vi "Labview to arduino VISA.vi"() -> ()   [LabVIEW 2012]
uses:
  <vilib>/Instr/_visa.llb/VISA Configure Serial Port (Instr).vi
panel:
  out "Meter":dbl(knob) scale=0.0..1024.0
  out "Waveform Chart":dbl(graph)
  out "Extracted Value":dbl
  in  "All Off":bool
  in  "LED 3":bool
  in  "LED 2":bool
  in  "LED 1":bool
  in  "Slide":dbl(slide) step=1.0 scale=0.0..1.0 scale format="%#_1g"
  out "Bytes Read":u32
  out "Raw Output":string="\n"
  in  "Input":refnum<visa-resource-name>="COM1"
  in  "Baud Rate":u32=9600
  # "Read"
  # "Write"
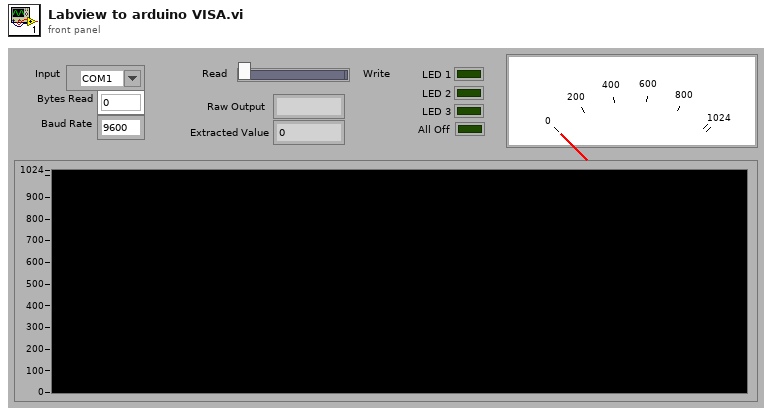
[diagram p1: front panel]
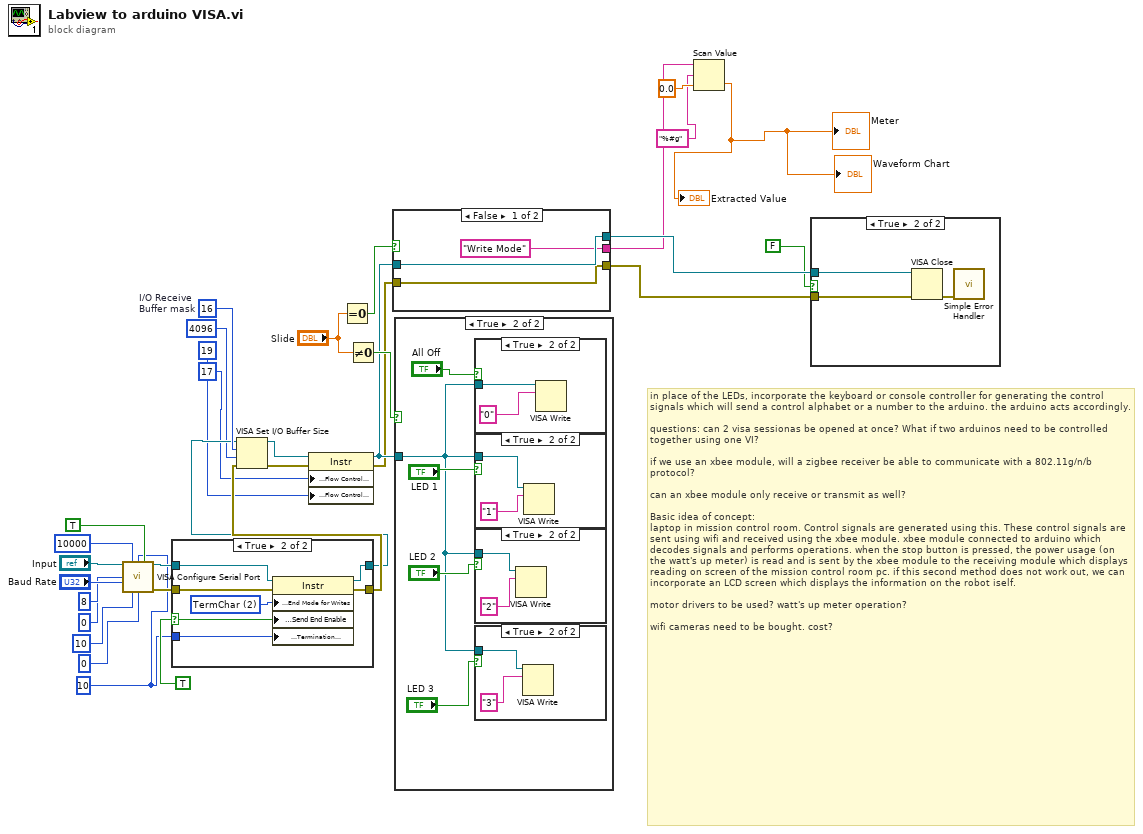
[diagram p0: block diagram]
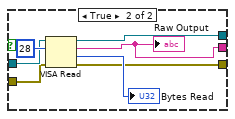
[diagram p8: hidden frame]
diagram:
  w13 = u8 10
  w30 = u16 16  # I/O Receive Buffer mask
  # "in place of the LEDs, incorporate the keyboard or console controller for generating the control signals which will send a control alphabet or a number to the arduino. the arduino acts accordingly.  \n\nquestions: can 2 visa sessionas be opened at once? What if two arduinos need to be controlled together using one VI?\n\nif we use an xbee module, will a zigbee receiver be able to communicate with a 802.11g/n/b protocol?\n\ncan an xbee module only receive or transmit as well?\n\nBasic idea of concept:\nlaptop in mission control room. Control signals are generated using this. These control signals are sent using wifi and received using the xbee module. xbee module connected to arduino which decodes signals and performs operations. when the stop button is pressed, the power usage (on the watt's up meter) is read and is sent by the xbee module to the receiving module which displays reading on screen of the mission control room pc. if this second method does not work out, we can incorporate an LCD screen which displays the information on the robot iself. \n\nmotor drivers to be used? watt's up meter operation? \n\nwifi cameras need to be bought. cost?"
  n1 = call-poly "VISA Configure Serial Port"("VISA resource name"="Input", "timeout (10sec)"=u32 10000, "termination char\n(0xA = '\\n' = LF)"=w13, "Enable Termination\nChar (T)"=TRUE, "baud rate (9600)"="Baud Rate", "data bits (8)"=u16 8, "parity (0:none)"=u16 0, "stop bits (10: 1 bit)"=u16 10, "flow control (0:none)"=u16 0) -> ("VISA resource name out"=w24:refnum<visa-resource-name>, "error out"=w27:errorcluster)  [unwired: 1 in, 4 out]
  n2 = case shown="True" TRUE {
    selector: TRUE -> [_ w35]
    tunnel: w24 -> [w33 w41]
    tunnel: w27 -> [w34 w40]
    tunnel: [w33 w39] -> w25
    tunnel: [w34 w38] -> w26
    tunnel: w13 -> [_ w36]
    frame False {
    }
    frame True {
      w37 = u16 2 items=["None", "LastBit", "TermChar", "Break"] ("Serial Settings:Serial End Mode for Writes")
      n3 = property class="Instr"(reference=w41, error in=w40, "Serial Settings:End Mode for Writes"=w37, "Message Based Settings:Send End Enable"=w35, "Message Based Settings:Termination Character"=w36) -> (reference out=w39:refnum<visa-resource-name>, error out=w38:errorcluster)
    }
  }
  n4 = VISA Set I/O Buffer Size(VISA resource name=w25, mask (16)=w30, size (4096)=u32 4096, error in (no error)=w26) -> (VISA resource name out=w29:refnum<visa-resource-name>, error out=w28:errorcluster)
  n5 = property class="Instr"(reference=w29, error in=w28, "Serial Settings:Flow Control XON Character"=u8 17, "Serial Settings:Flow Control XOFF Character"=u8 19) -> (reference out=w9:refnum<visa-resource-name>, error out=w5:errorcluster)
  n6 = Equal To 0?(x="Slide") -> (x = 0?=w12:bool)
  n7 = Not Equal To 0?(x="Slide") -> (x != 0?=w11:bool)
  n8 = case shown="False" w12 {
    tunnel: w9 -> [w44 w49]
    tunnel: [w44 w48] -> w8
    tunnel: [w43 w47] -> w7
    tunnel: ["Write Mode" w46] -> w6
    tunnel: w5 -> [w43 w45]
    frame False {
    }
    frame True {
      n9 = VISA Read(VISA resource name=w49, byte count=u32 28, error in (no error)=w45) -> (VISA resource name out=w48:refnum<visa-resource-name>, read buffer=w46:string, return count=→"Bytes Read":u32, error out=w47:errorcluster)
      "Raw Output" <- w46
    }
  }
  n10 = case shown="True" w11 {
    tunnel: w9 -> [_ w52]
    frame False {
    }
    frame True {
      n11 = case shown="True" "All Off" {
        tunnel: w52 -> [_ w63]
        frame False {
        }
        frame True {
          n12 = VISA Write(VISA resource name=w63, write buffer="0") -> ()  [unwired: 1 in, 3 out]
        }
      }
      n13 = case shown="True" "LED 1" {
        tunnel: w52 -> [_ w61]
        frame False {
        }
        frame True {
          n14 = VISA Write(VISA resource name=w61, write buffer="1") -> ()  [unwired: 1 in, 3 out]
        }
      }
      n15 = case shown="True" "LED 2" {
        tunnel: w52 -> [_ w59]
        frame False {
        }
        frame True {
          n16 = VISA Write(VISA resource name=w59, write buffer="2") -> ()  [unwired: 1 in, 3 out]
        }
      }
      n17 = case shown="True" "LED 3" {
        tunnel: w52 -> [_ w57]
        frame False {
        }
        frame True {
          n18 = VISA Write(VISA resource name=w57, write buffer="3") -> ()  [unwired: 1 in, 3 out]
        }
      }
    }
  }
  n19 = Scan Value(string=w6, format string="%#g", default (0 dbl)=0.0) -> (value=→"Extracted Value" →"Waveform Chart" →"Meter":dbl)  [unwired: 1 out]
  n20 = case shown="True" FALSE {
    tunnel: w8 -> [_ w66]
    tunnel: w7 -> [_ w65]
    frame False {
    }
    frame True {
      n21 = VISA Close(VISA resource name=w66, error in (no error)=w65) -> (error out=w67:errorcluster)
      n22 = call <vilib>:"Simple Error Handler.vi"("error in (no error)"=w67) -> ()  [unwired: 1 in, 8 out]
    }
  }
